vi "Destroy User Events.vi"(11 "UI Template in":refnum<class "Measurement GEN.lvclass">) -> (3 "UI Template out":refnum<class "Measurement GEN.lvclass">)   [LabVIEW 2020, in "Measurement GEN.lvlib" / "Measurement GEN.lvclass"]
uses:
  Measurement GEN.lvclass
  Measurement GEN.lvclass/Measurement GEN.ctl
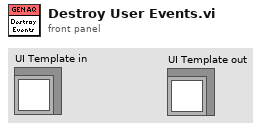
[diagram p1: front panel]
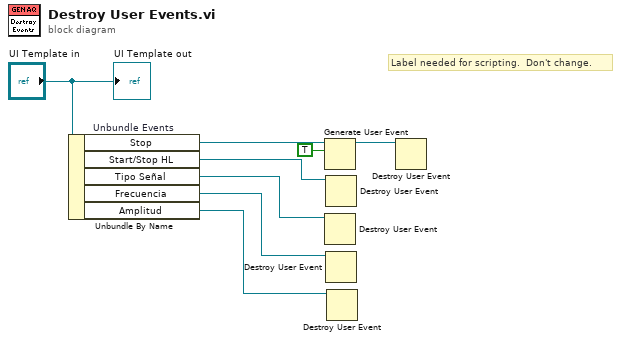
[diagram p0: block diagram]
diagram:
  # "Label needed for scripting.  Don't change."
  n1 = Unbundle By Name "Unbundle Events"("UI Template in") -> ("Stop"=w6:refnum<user-event>, "Start/Stop HL"=w4:refnum<user-event>, "Tipo Señal"=w3:refnum<user-event>, "Frecuencia"=w2:refnum<user-event>, "Amplitud"=w1:refnum<user-event>)
  n2 = Generate User Event(user event=w6, event data cluster=TRUE ("event data")) -> (user event out=w7:refnum<user-event>)  [unwired: 2 in, 1 out]
  n3 = Destroy User Event(user event=w3) -> ()  [unwired: 1 in, 1 out]
  n4 = Destroy User Event(user event=w4) -> ()  [unwired: 1 in, 1 out]
  n5 = Destroy User Event(user event=w2) -> ()  [unwired: 1 in, 1 out]
  n6 = Destroy User Event(user event=w1) -> ()  [unwired: 1 in, 1 out]
  n7 = Destroy User Event(user event=w7) -> ()  [unwired: 1 in, 1 out]
  "UI Template out" <- "UI Template in"
